vi "Run IR_READ_WRITE.vi"() -> ()   [LabVIEW 2014]
panel:
  in  "Number of files to read":dbl=1.0
  out "averagePeaksStr":string
  out "averagePeaks":dbl[](array[numeric])
  out "error out":errorcluster
  out "Is SS?":bool
  in  "Excel Sheet Name":string="Cont_Res_Time_Ramp_Results"
  in  "Peak Heights(comma separated)":string="780"
  in  "Report File":string="C:\\Users\\Admin\\Documents\\Kosi\\Comprehensive_Labview_Report_Template.xlsx"
  in  "IR Read Dir.":string="C:\\Users\\Admin\\Documents\\Kosi\\old_ramp_data"
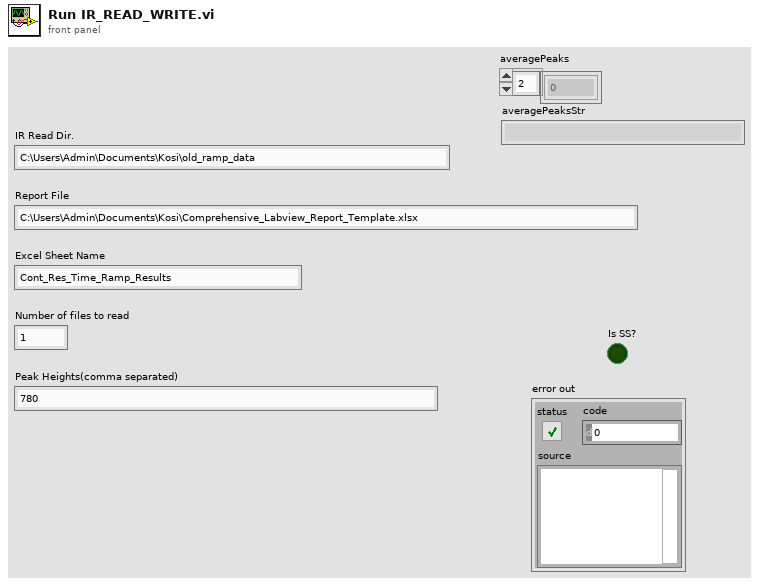
[diagram p1: front panel]
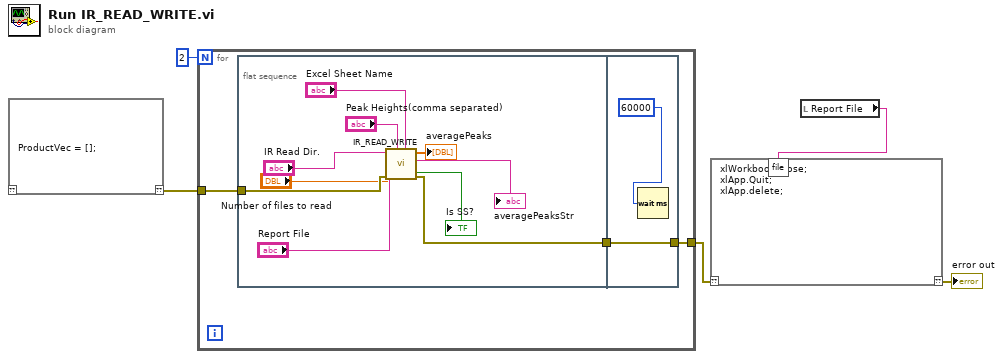
[diagram p0: block diagram]
diagram:
  n1 = script code="ProductVec = [];"() -> ("??"=w2:errorcluster)  [unwired: 1 in]
  n2 = for {
    N: 2 -> [_]
    tunnel: [w7] -> w3
    tunnel: w2 -> [w8]
    n3 = flat-sequence {
      tunnel: w8 -> [w13]
      tunnel: [w12] -> w6
      tunnel: [w20] -> w7
      tunnel: w6 -> [w20]
      frame #0 {
        n4 = call "IR_READ_WRITE.vi"("Excel Sheet Name"="Excel Sheet Name", "Peak Heights(comma separated)"="Peak Heights(comma separated)", "error constant"=w13, "Number of files to read"="Number of files to read", "Report temp"="Report File", "IR Read Dir."="IR Read Dir.") -> ("error constant 2"=w12:errorcluster, "averagePeaksStr"=→"averagePeaksStr":string, "averagePeaks"=→"averagePeaks":dbl[], "Is SS?"=→"Is SS?":bool)  [unwired: 2 in]
      }
      frame #1 {
        n5 = Wait (ms)(milliseconds to wait=u32 60000) -> ()  [unwired: 1 out]
      }
    }
  }
  n6 = local read "Report File"() -> (w4:string)
  n7 = script code="xlWorkbook.Close;\nxlApp.Quit;\nxlApp.delete;"("??"=w3, "file"=w4) -> ("??"=→"error out":errorcluster)
